vi "Report Cal Measured Freq Dll.vi"(0 "CART TCP Connection In":refnum<k5>, 5 "XtalCalChain":u32, 7 "XtalCalVal":dbl) -> (4 "CART TCP Connection Out":refnum<k5>, 6 "StatusIsFalse":i16)   [LabVIEW 2011]
uses:
  WLAN/UUT/QCA/NART Constants.vi
panel:
  out "Command Sent":string
  out "TCP Messages":string[](array[string])
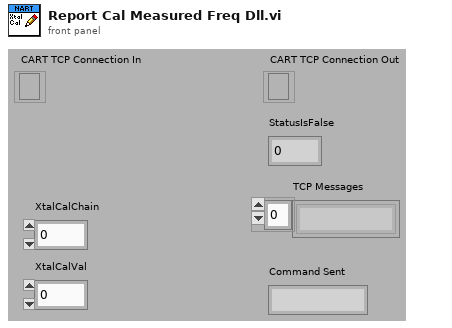
[diagram p1: front panel]
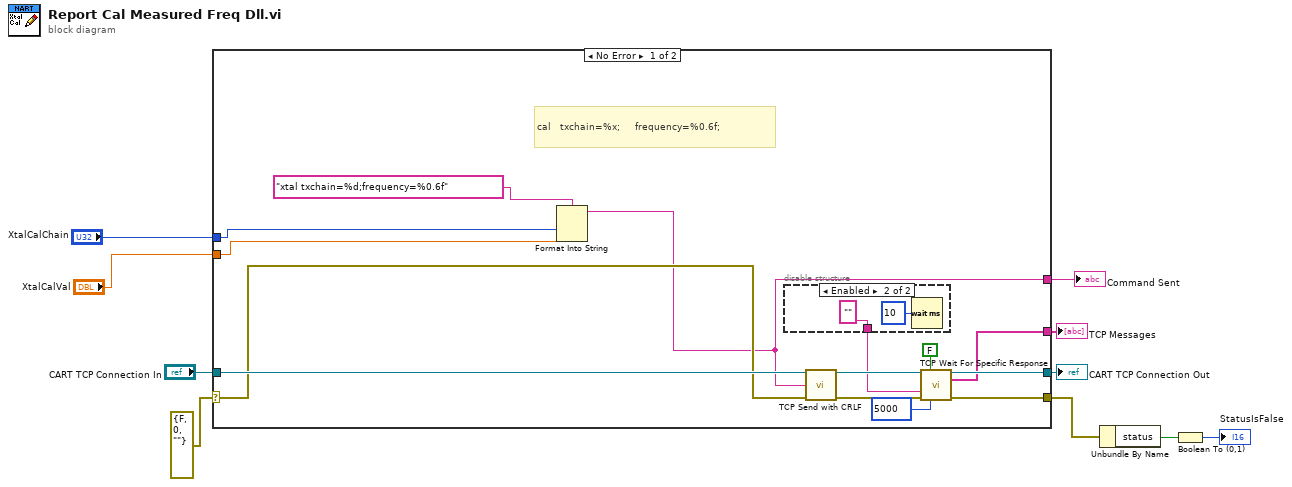
[diagram p0: block diagram]
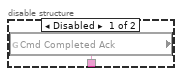
[diagram p2: hidden frame]
diagram:
  n1 = case shown="No Error" errorcluster {"status"=FALSE, "code"=0, "source"=""} ("error in (no error)") {
    selector: errorcluster {"status"=FALSE, "code"=0, "source"=""} ("error in (no error)") -> [w23 w29]
    tunnel: [w20 w29] -> w5
    tunnel: "CART TCP Connection In" -> [w24 w28]
    tunnel: [w21 w28] -> w8
    tunnel: [w17 _] -> w7
    tunnel: [w11 _] -> w6
    tunnel: "XtalCalChain" -> [w14 _]
    tunnel: "XtalCalVal" -> [w13 _]
    frame No Error {
      # "cal   txchain=%x;     frequency=%0.6f;"
      n2 = Format Into String(format string="xtal txchain=%d;frequency=%0.6f", w14, w13) -> (resulting string=w11:string)  [unwired: 2 in, 1 out]
      n3 = disable-structure shown="Enabled" {
        disable-tunnel: [w25 "" ("Expected Message Start (\"\":any)")] -> w15
        frame Disabled {
          n4 = global read "NART Constants.vi" "Cmd Completed Ack"() -> (w25:string)
        }
        frame Enabled {
          n5 = Wait (ms)(milliseconds to wait=u32 10) -> ()  [unwired: 1 out]
        }
      }
      n6 = call "TCP Send with CRLF.vi"("CART TCP Connection"=w24, "data in"=w11, "error IO"=w23) -> ("CART TCP Connection Out"=w22:refnum<k5>, "error out"=w19:errorcluster)  [unwired: 11 in]
      n7 = call "TCP Wait For Specific Response.vi"("TCP Connection In"=w22, "Next response (t)"=FALSE, "Expected Message Start (\"\":any)"=w15, "error in"=w19, "Timeout (250 ms)"=5000) -> ("TCP Connection Out"=w21:refnum<k5>, "TCP Messages"=w17:string[], "error out"=w20:errorcluster)  [unwired: 7 in, 1 out]
    }
    frame Error {
    }
  }
  "CART TCP Connection Out" <- w8
  "TCP Messages" <- w7
  "Command Sent" <- w6
  n8 = Unbundle By Name(w5) -> ("status"=w3:bool)
  n9 = Boolean To (0,1)(Boolean=w3) -> (0, 1=→"StatusIsFalse":i16)
